vi "moveArm (SubVI).vi"(11 "Arm stoke(mm)":sgl) -> (3 "Arm angle(deg)":sgl)   [LabVIEW 2020]
uses:
  <vilib>/imath/engines/lvmath2/RunTimeEngine/NodeEndStatement/NIMS_NodeEndStatement_Output.vi
  <instcachedir>/0/NIMS_NodeEndStatement_Output_53EC0D466D134D7ABD903AC30B43404B.lvgen/NIMS_NodeEndStatement_Output_53EC0D466D134D7ABD903AC30B43404B_009.vi
  <vilib>/imath/engines/lvmath2/RunTimeEngine/ErrorHandling/NIMS_Finalize Error.vi
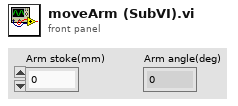
[diagram p1: front panel]
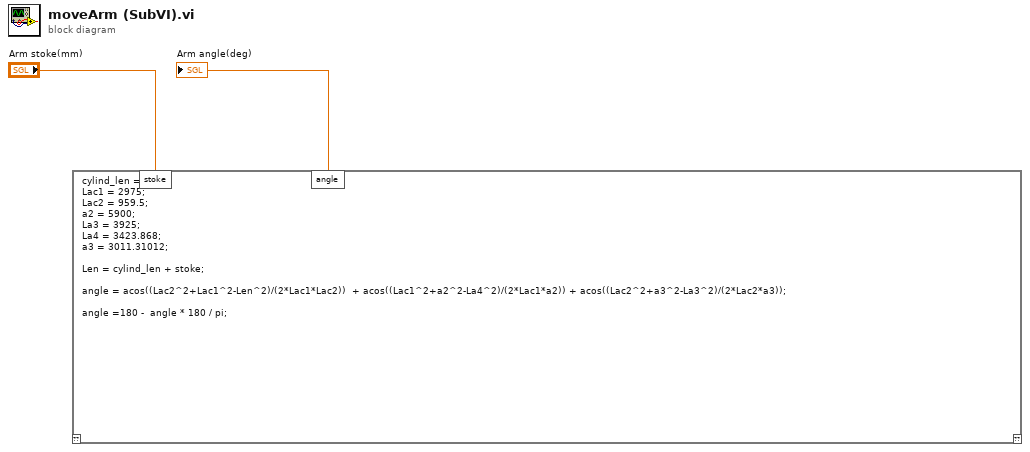
[diagram p0: block diagram]
diagram:
  n1 = mathscript code="cylind_len = 2183;\nLac1 = 2975;\nLac2 = 959.5;\na2 = 5900;\nLa3 = 3925;\nLa4 = 3423.868;\na3 = 3011.31012;\n\nLen = cylind_len + stoke;\n\nangle = acos((Lac2^2+Lac1^2-Len^2)/(2*Lac1*Lac2))  + acos((Lac1^2+a2^2-La4^2)/(2*Lac1*a2)) + acos((Lac2^2+a3^2-La3^2)/(2*Lac2*a3));\n\nangle =180 -  angle * 180 / pi;"("stoke"="Arm stoke(mm)") -> ("angle"=→"Arm angle(deg)":cdb)  [unwired: 1 in, 1 out]
